vi "FindingMultiplesSize.vi"(8 "error in (no error)":errorcluster, 11 "TableLogger_Actor in":refnum<class "TableLogger_Actor.lvclass">) -> (0 "error out":errorcluster, 2 "MaxDBSize?T":bool, 3 "TableLogger_Actor out":refnum<class "TableLogger_Actor.lvclass">)   [LabVIEW 2014, in "TableLogger_Actor.lvlib" / "TableLogger_Actor.lvclass"]
doc: "This VI checks the size of a dB source file path to take backup, whenever the DB backup on size multiples (in bytes) has reached."
uses:
  TableLogger_Actor.lvclass
  TableLogger_Actor.lvclass/TableLogger_Actor.ctl
  <vilib>/ActorFramework/Message Enqueuer/Message Priority.ctl
  <vilib>/ActorFramework/Actor/Actor.lvclass/Actor.ctl
  <vilib>/ActorFramework/Message Enqueuer/Message Enqueuer.lvclass/Message Enqueuer.ctl
  <vilib>/ActorFramework/Message Enqueuer/Init from Existing Queue.vi
  <vilib>/ActorFramework/Message Enqueuer/Enqueue.vi
  <vilib>/ActorFramework/Message Priority Queue/Priority Enqueue.vi
  <vilib>/ActorFramework/Message Enqueuer/Message Enqueuer.lvclass
  TableLogger_Actor Messages/BackupDB Msg/BackupDB Msg.lvclass
  <vilib>/ActorFramework/Actor/Actor.lvclass
panel:
  # "This VI checks the size of a dB source file path to take backup, whenever the DB backup on size multiples (in bytes) has reached."
  # "Connector Pane"
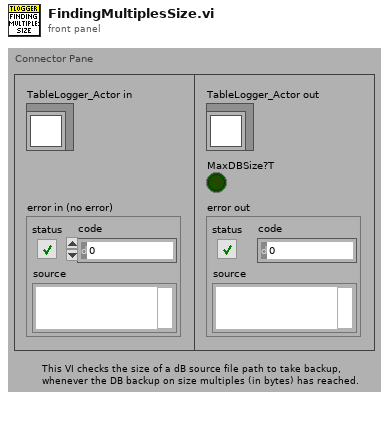
[diagram p1: front panel]
types:
  T1 = typedef "Actor Framework.lvlib/Message Enqueuer.lvclass/Message Priority.ctl" = enum16{"Low", "Normal", "High"}
  T2 = typedef "File Info Record__ogtk.ctl" = cluster{"type":string, "creator":string, "permissions":i32, "data size":i32, "res size":i32, "creation date":u32, "modification date":u32, "bFolder":bool, "bInvisible":bool, "location":cluster{"vertical":i16, "horizontal":i16}, "owner":string, "group":string}
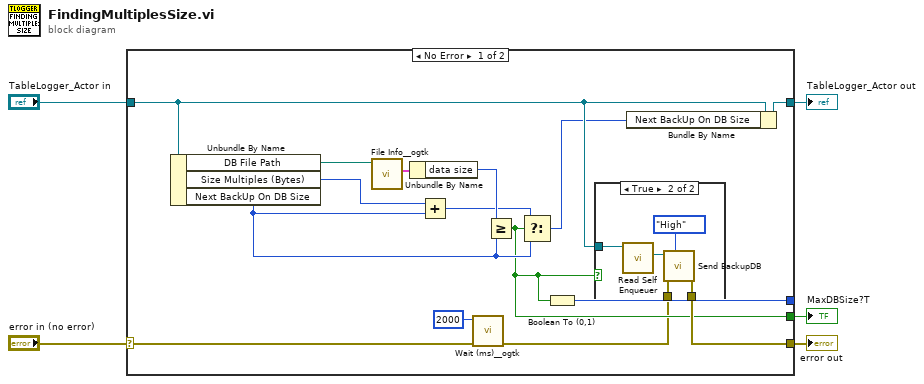
[diagram p0: block diagram]
diagram:
  n1 = case shown="No Error" "error in (no error)" {
    selector: "error in (no error)" -> [w20 w27]
    tunnel: [w18 w27] -> w5
    tunnel: [w17 w28] -> w3
    tunnel: "TableLogger_Actor in" -> [w16 w28]
    tunnel: [w9 _] -> w1
    tunnel: [w8 _] -> _
    frame No Error {
      n2 = Unbundle By Name(w16) -> ("DB File Path"=w19:path, "Size Multiples (Bytes)"=w13:i32, "Next BackUp On DB Size"=w10:i32)
      n3 = call <userlib>:"File Info__ogtk.vi"("file"=w19) -> ("file info"=w14:T2)  [unwired: 5 in, 2 out]
      n4 = Unbundle By Name(w14) -> ("data size"=w15:i32)
      n5 = Add(x=w13, y=w10) -> (x+y=w12:i32)
      n6 = call <userlib>:"Wait (ms)__ogtk.vi"("error in (no error)"=w20, "milliseconds to wait"=u32 2000) -> ("error out"=w7:errorcluster)  [unwired: 8 in, 1 out]
      n7 = Greater Or Equal?(x=w15, y=w10) -> (x >= y?=w9:bool)
      n8 = Select(t=w12, s=w9, f=w10) -> (s? t:f=w11:i32)
      n9 = Boolean To (0,1)(Boolean=w9) -> (0, 1=w8:i16)
      n10 = case shown="True" w9 {
        tunnel: w16 -> [_ w25]
        tunnel: w7 -> [w21 w24]
        tunnel: [w21 w23] -> w18
        frame False {
        }
        frame True {
          n11 = call <vilib>:"Read Self Enqueuer.vi"("Actor"=w25) -> ("Self Enqueuer"=w26:refnum<class "Message Enqueuer.lvclass">)  [unwired: 10 in]
          n12 = call "Send BackupDB.vi"("Message Priority (Normal)"=Message_Priority."High", "error in (no error)"=w24, "Message Enqueuer"=w26) -> ("error out"=w23:errorcluster)  [unwired: 7 in, 1 out]
        }
      }
      n13 = Bundle By Name(cluster=w16, "Next BackUp On DB Size"=w11) -> (w17:refnum<class "TableLogger_Actor.lvclass">)
    }
    frame Error {
    }
  }
  "TableLogger_Actor out" <- w3
  "error out" <- w5
  "MaxDBSize?T" <- w1
